vi "Day 1.1 - Most Calories.vi"(11 "input":u64[](array[numeric])) -> (3 "output":u64)   [LabVIEW 2021]
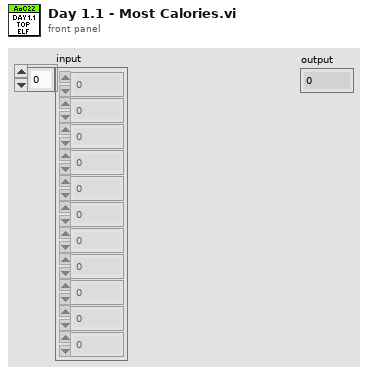
[diagram p1: front panel]
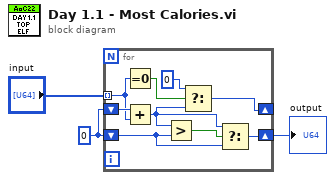
[diagram p0: block diagram]
diagram:
  w2 = u64 0
  n1 = for {
    tunnel: "input" -> [w11] mode=indexing
    shift-right: [w9] -> _
    shift-left: w2 -> [w12]
    shift-right: [w5] -> w1
    shift-left: w2 -> [w4]
    n2 = Equal To 0?(x=w11) -> (x = 0?=w10:bool)
    n3 = Add(x=w12, y=w11) -> (x+y=w6:u64)
    n4 = Greater?(x=w6, y=w4) -> (0:w7:bool)
    n5 = Select(t=0, s=w10, f=w6) -> (s? t:f=w9:u64)
    n6 = Select(t=w6, s=w7, f=w4) -> (s? t:f=w5:u64)
  }
  "output" <- w1
